vi "Get Menu Items.vi"(8 "error in (no error)":errorcluster, 9 "GUID":string, 10 "Item Ref":T1 format="%.0x", 11 "System Explorer Dispatcher Implementation in":refnum<class "System Explorer Dispatcher.lvclass">) -> (0 "error out":errorcluster, 2 "Menu Items":cluster{"Name":string, "Enabled?":bool}[](array[cluster]), 3 "System Explorer Dispatcher Implementation out":refnum<class "System Explorer Dispatcher.lvclass">)   [LabVIEW 2020, in "AIM ARINC 664 System Explorer.lvlib" / "Implementation.lvlib" / "System Explorer Dispatcher.lvclass"]
uses:
  System Explorer Dispatcher.lvclass
  <vilib>/NI VeriStand/Custom Device API/Custom Device Item Ref.ctl
  Scripting/Constants.vi
  Scripting/AIM ARINC 664 Scripting.lvlib
  <vilib>/NI VeriStand/Custom Device API/Custom Device API.lvlib
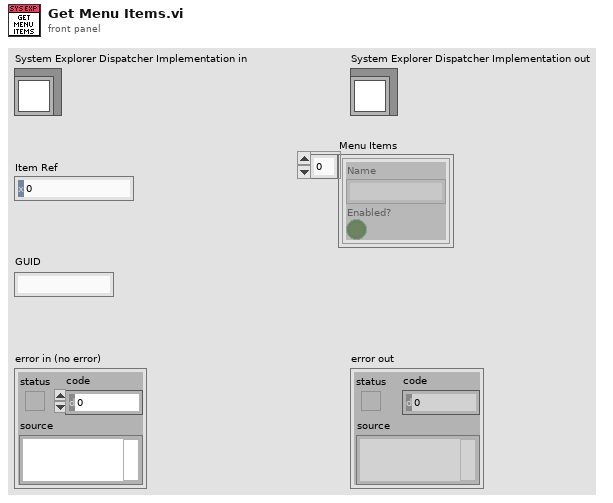
[diagram p1: front panel]
types:
  T1 = typedef "Custom Device API.lvlib/Custom Device Item Ref.ctl" = u64
  T2 = map{string, cluster{"Tag":string, "Enabled?":bool}[]}
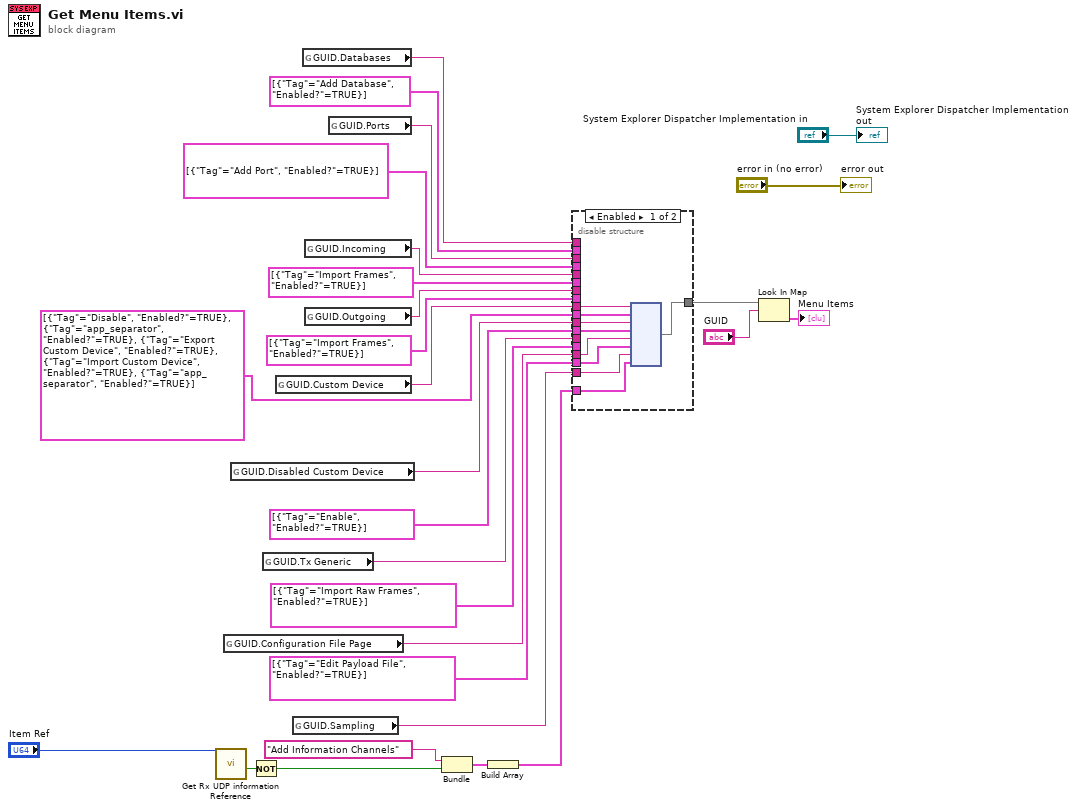
[diagram p0: block diagram]
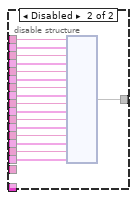
[diagram p2: hidden frame]
diagram:
  n1 = call "Get Rx UDP information Reference.vi"("custom device ref"="Item Ref") -> ("found?"=w5:bool)  [unwired: 8 in, 2 out]
  n2 = global read "Constants.vi" "GUID.Configuration File Page"() -> (w9:string)
  n3 = global read "Constants.vi" "GUID.Disabled Custom Device"() -> (w18:string)
  n4 = Not(x=w5) -> (.not. x?=w4:bool)
  n5 = global read "Constants.vi" "GUID.Tx Generic"() -> (w11:string)
  n6 = global read "Constants.vi" "GUID.Custom Device"() -> (w19:string)
  n7 = global read "Constants.vi" "GUID.Sampling"() -> (w1:string)
  n8 = global read "Constants.vi" "GUID.Databases"() -> (w23:string)
  n9 = global read "Constants.vi" "GUID.Incoming"() -> (w21:string)
  n10 = global read "Constants.vi" "GUID.Outgoing"() -> (w20:string)
  n11 = global read "Constants.vi" "GUID.Ports"() -> (w22:string)
  n12 = Bundle("Tag"="Add Information Channels", w4) -> (w3:cluster{"Tag":string, bool})  [unwired: 1 in]
  n13 = Build Array(w3) -> (w2:cluster{"Tag":string, bool}[])
  n14 = disable-structure shown="Enabled" {
    disable-tunnel: [w37 w54] -> w26
    disable-tunnel: w23 -> [_ w53]
    disable-tunnel: w22 -> [_ w52]
    disable-tunnel: w21 -> [_ w51]
    disable-tunnel: w20 -> [_ w50]
    disable-tunnel: w19 -> [w36 w49]
    disable-tunnel: w18 -> [w35 w48]
    disable-tunnel: cluster{"Tag":string, "Enabled?":bool}[] [{"Tag"="Add Database", "Enabled?"=TRUE}] ("Menu Items") -> [_ w47]
    disable-tunnel: cluster{"Tag":string, "Enabled?":bool}[] [{"Tag"="Add Port", "Enabled?"=TRUE}] ("Menu Items") -> [_ w46]
    disable-tunnel: cluster{"Tag":string, "Enabled?":bool}[] [{"Tag"="Import Frames", "Enabled?"=TRUE}] ("Menu Items") -> [_ w45]
    disable-tunnel: cluster{"Tag":string, "Enabled?":bool}[] [{"Tag"="Import Frames", "Enabled?"=TRUE}] ("Menu Items") -> [_ w44]
    disable-tunnel: cluster{"Tag":string, "Enabled?":bool}[] [{"Tag"="Enable", "Enabled?"=TRUE}] ("Menu Items") -> [w34 w43]
    disable-tunnel: cluster{"Tag":string, "Enabled?":bool}[] [{"Tag"="Disable", "Enabled?"=TRUE}, {"Tag"="app_separator", "Enabled?"=TRUE}, {"Tag"="Export Custom Device", "Enabled?"=TRUE}, {"Tag"="Import Custom Device", "Enabled?"=TRUE}, {"Tag"="app_separator", "Enabled?"=TRUE}] ("Menu Items") -> [w33 w42]
    disable-tunnel: w11 -> [_ w41]
    disable-tunnel: cluster{"Tag":string, "Enabled?":bool}[] [{"Tag"="Import Raw Frames", "Enabled?"=TRUE}] ("value") -> [_ w40]
    disable-tunnel: w9 -> [w32 w39]
    disable-tunnel: cluster{"Tag":string, "Enabled?":bool}[] [{"Tag"="Edit Payload File", "Enabled?"=TRUE}] ("value") -> [w31 w38]
    disable-tunnel: w2 -> [w30 _]
    disable-tunnel: w1 -> [w29 _]
    frame Enabled {
      n15 = node(w36, w33, w35, w34, w32, w31, w29, w30) -> (w37:T2)
    }
    frame Disabled {
      n16 = node(w53, w47, w52, w46, w51, w45, w50, w44, w49, w42, w48, w43, w41, w40, w39, w38) -> (w54:T2)
    }
  }
  n17 = Look In Map(map=w26, key="GUID") -> (value=→"Menu Items":cluster{"Tag":string, "Enabled?":bool}[])  [unwired: 1 in, 1 out]
  "error out" <- "error in (no error)"
  "System Explorer Dispatcher Implementation out" <- "System Explorer Dispatcher Implementation in"
